vi "u2q_big.vi"(1 "In":u16[][](array[numeric]), 2 "U_Ch":u16[](array[numeric]), 3 "Ch":u16) -> (0 "Out":i32[][](array[numeric]))   [LabVIEW 2010]
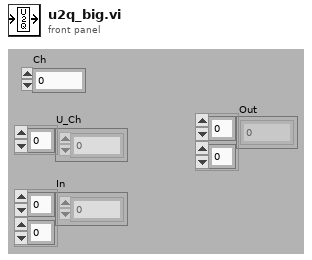
[diagram p1: front panel]
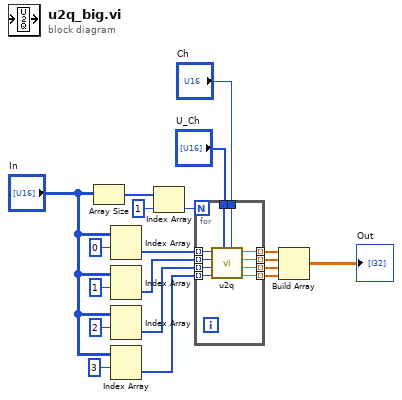
[diagram p0: block diagram]
diagram:
  n1 = Array Size(array="In") -> (size(s)=w2:i32[])
  n2 = Index Array(array="In", index (row)=0 ("index")) -> (element=w1:u16[])  [unwired: 1 in]
  n3 = Index Array(array="In", index (row)=1 ("index")) -> (element=w9:u16[])  [unwired: 1 in]
  n4 = Index Array(array="In", index (row)=2 ("index")) -> (element=w10:u16[])  [unwired: 1 in]
  n5 = Index Array(array="In", index (row)=3 ("index")) -> (element=w11:u16[])  [unwired: 1 in]
  n6 = Index Array(array=w2, index=1) -> (element=w4:i32)
  n7 = for {
    N: w4 -> [_]
    tunnel: w1 -> [w29] mode=indexing
    tunnel: w9 -> [w28] mode=indexing
    tunnel: w10 -> [w27] mode=indexing
    tunnel: w11 -> [w26] mode=indexing
    tunnel: [w25] -> w12 mode=indexing
    tunnel: [w24] -> w13 mode=indexing
    tunnel: [w23] -> w14 mode=indexing
    tunnel: [w22] -> w15 mode=indexing
    tunnel: "U_Ch" -> [w21]
    tunnel: "Ch" -> [w20]
    n8 = call "u2q.vi"("Ch"=w20, "U_ch"=w21, "x4"=w26, "x3"=w27, "x2"=w28, "x1"=w29) -> ("y4"=w22:dbl, "y3"=w23:dbl, "y2"=w24:dbl, "y1"=w25:dbl)
  }
  n9 = Build Array(w12, w13, w14, w15) -> (→"Out":dbl[][])
